vi "warten auf Stein vom Förderband.vi"(8 "error in (no error)":errorcluster caption="Fehler (Eingang, kein Fehler)", 9 "Digital_Input":T1(ring), 10 "Module":T2(ring), 11 "Device ID":T3(ring)) -> (0 "error out":errorcluster caption="Fehler (Ausgang)", 3 "Device ID Out":T3(ring))   [LabVIEW 2010]
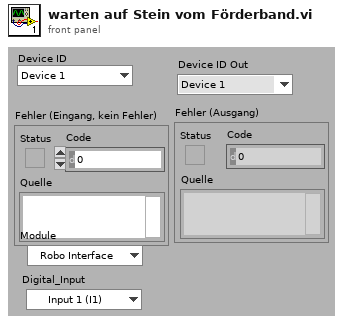
[diagram p1: front panel]
types:
  T1 = enum8{"Input 1 (I1)", "Input 2 (I2)", "Input 3 (I3)", "Input 4 (I4)", "Input 5 (I5)", "Input 6 (I6)", "Input 7 (I7)", "Input 8 (I8)"}
  T2 = enum8{"Robo Interface", "Extension 1", "Extension 2", "Extension 3"}
  T3 = enum16{"Device 1", "Device 2", "Device 3", "Device 4", "Device 5", "Device 6", "Device 7", "Device 8"}
  T4 = enum8{"Goes High", "Goes Low", "Goes High or Low"}
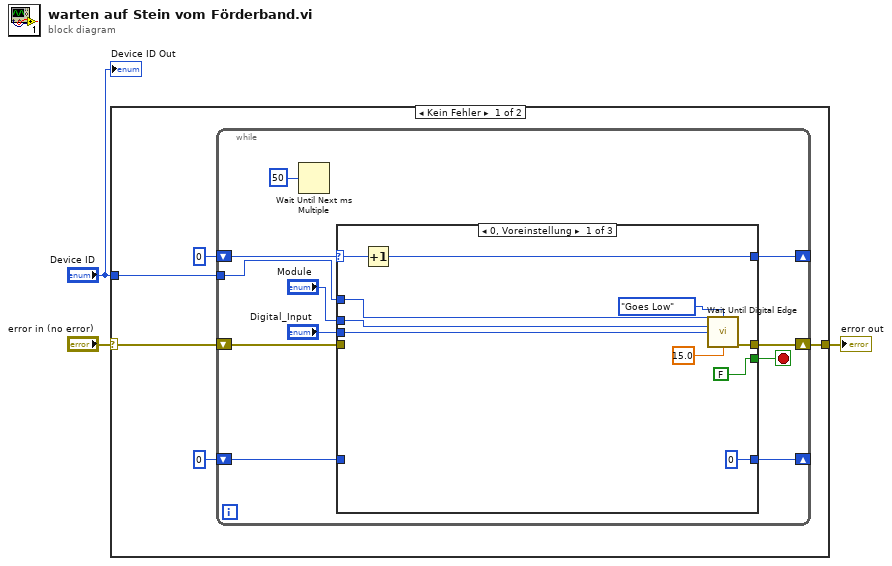
[diagram p0: block diagram]
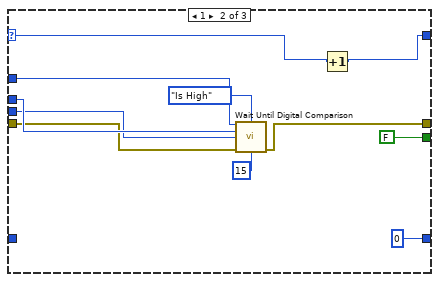
[diagram p2: hidden frame]
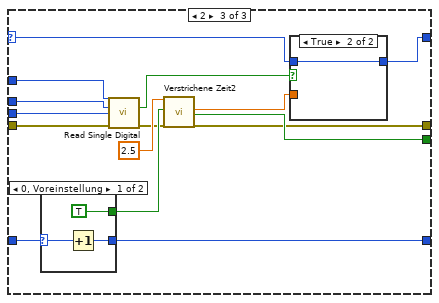
[diagram p3: hidden frame]
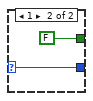
[diagram p4: hidden frame]
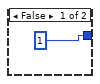
[diagram p5: hidden frame]
diagram:
  n1 = case shown="Kein Fehler" "error in (no error)" {
    selector: "error in (no error)" -> [w8 w63]
    tunnel: [w7 w63] -> w2
    tunnel: "Device ID" -> [w6 _]
    frame No Error {
      n2 = while {
        shift-right: [w14] -> w7
        shift-left: w8 -> [w15]
        tunnel: w6 -> [w16]
        shift-right: [w11] -> _
        shift-left: 0 -> [w19]
        shift-right: [w9] -> _
        shift-left: 0 -> [w10]
        stop <- w18 stop-if-true
        n3 = Wait Until Next ms Multiple(millisecond multiple=50) -> ()  [unwired: 1 out]
        n4 = case shown="0, Voreinstellung" w19 {
          selector: w19 -> [w21 w30 w52]
          tunnel: [FALSE ("Time has Elapsed") FALSE w46] -> w18
          tunnel: w16 -> [w27 w38 w45]
          tunnel: w15 -> [_ w35 w54]
          tunnel: [w22 w34 w42] -> w14
          tunnel: "Module" -> [w26 w37 w44]
          tunnel: "Digital_Input" -> [w25 w36 w43]
          tunnel: [w20 w31 w53] -> w11
          tunnel: w10 -> [_ _ w49]
          tunnel: [0 0 w47] -> w9
          frame 0, Default {
            n5 = Increment(x=w21) -> (x+1=w20:i32)
            n6 = call "Wait Until Digital Edge.vi"("Device ID"=w27, "Wait Until"=T4."Goes Low", "Module"=w26, "Digital_Input"=w25, "Time Out (10)"=15.0) -> ("error out"=w22:errorcluster)  [unwired: 1 in, 9 out]
          }
          frame 1 {
            n7 = call "Wait Until Digital Comparison.vi"("Device ID"=w38, "Wait Until"=enum8{"Is High", "Is Low"}."Is High", "Module"=w37, "Digital_Input"=w36, "error in"=w35, "Time Out (10)"=15) -> ("error out"=w34:errorcluster)  [unwired: 9 out]
            n8 = Increment(x=w30) -> (x+1=w31:i32)
          }
          frame 2 {
            n9 = case shown="0, Voreinstellung" w49 {
              selector: w49 -> [w57 w59]
              tunnel: [TRUE FALSE] -> w48
              tunnel: [w56 w59] -> w47
              frame 0, Default {
                n10 = Increment(x=w57) -> (x+1=w56:i32)
              }
              frame 1 {
              }
            }
            n11 = call "Read Single Digital.vi"("Device ID"=w45, "Module"=w44, "Digital_Input"=w43, "error in"=w54) -> ("Value"=w55:bool, "error out"=w41:errorcluster)  [unwired: 10 out]
            n12 = call "Verstrichene Zeit2"("Time Target (s)"=2.5, "Reset"=w48, "error in (no error)"=w41) -> ("Elapsed Time (s)"=w51:dbl, "Time has Elapsed"=w46:bool, "error out"=w42:errorcluster)  [unwired: 2 in, 12 out]
            n13 = case shown="TRUE" w55 {
              tunnel: w51 -> [_ _]
              tunnel: [1 w62] -> w53
              tunnel: w52 -> [_ w62]
              frame False {
              }
              frame True {
              }
            }
          }
        }
      }
    }
    frame Error {
    }
  }
  "error out" <- w2
  "Device ID Out" <- "Device ID"
